vi "rotate.vi"(8 "error in (no error)":errorcluster, 10 "angle":dbl[unit], 11 "Image in":refnum<class "Image.lvclass">) -> (0 "error out":errorcluster, 3 "Image out":refnum<class "Image.lvclass">)   [LabVIEW 2010, in "Image.lvclass"]
uses:
  Image.lvclass
  storage_mode.ctl
  ErrorController/ErrorController/class_data.vi
  <vilib>/vision/NI_Vision_Development_Module.lvlib
  ErrorController/ErrorController/ErrorController.lvclass
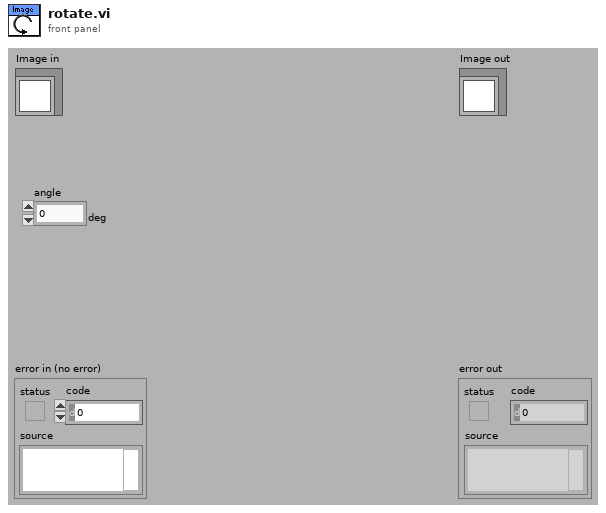
[diagram p1: front panel]
types:
  T1 = typedef "Image.lvclass/storage_mode.ctl" = enum16{"RAM", "disk"}
  T2 = typedef "IMAQ Image.ctl" = refnum<image>
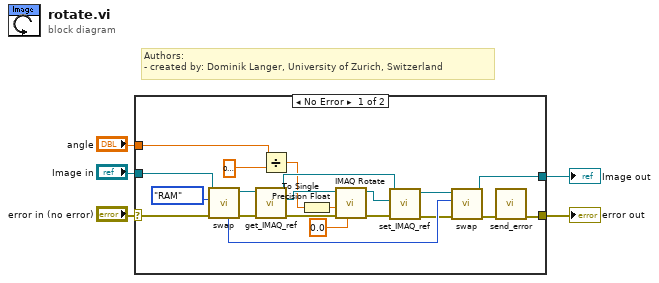
[diagram p0: block diagram]
diagram:
  # "Authors: \n- created by: Dominik Langer, University of Zurich, Switzerland"
  n1 = case shown="No Error" "error in (no error)" {
    selector: "error in (no error)" -> [w24 w28]
    tunnel: [w6 w28] -> w4
    tunnel: [w8 w27] -> w2
    tunnel: "Image in" -> [w10 w27]
    tunnel: "angle" -> [w9 _]
    frame No Error {
      n2 = call-dynamic "swap.vi"("error in (no error)"=w24, "storage type target"=storage_mode."RAM", "Image in"=w10) -> ("error out"=w23:errorcluster, "Image out"=w22:refnum<class "Image.lvclass">, "previous storage mode"=w25:T1)  [unwired: 6 out]
      n3 = call-dynamic "get_IMAQ_ref.vi"("error in (no error)"=w23, "Image.lvclass in"=w22) -> ("error out"=w21:errorcluster, "Image"=w20:T2, "Image.lvclass out"=w14:refnum<class "Image.lvclass">)  [unwired: 7 out]
      n4 = Divide(x=w9, y=dbl[unit] 0.017453292519943295 ("angle")) -> (x/y=w11:dbl)
      n5 = To Single Precision Float(number=w11) -> (single precision float=w18:sgl)
      n6 = call "IMAQ Rotate"("Replace Value"=sgl 0.0, "error in (no error)"=w21, "Angle (degrees)"=w18, "Image Src"=w20) -> ("error out"=w16:errorcluster, "Image Dst Out"=w15:T2)  [unwired: 4 in, 2 out]
      n7 = call-dynamic "set_IMAQ_ref.vi"("error in (no error)"=w16, "Image"=w15, "Image.lvclass in"=w14) -> ("error out"=w13:errorcluster, "Image.lvclass out"=w12:refnum<class "Image.lvclass">)  [unwired: 7 out]
      n8 = call-dynamic "swap.vi"("error in (no error)"=w13, "storage type target"=w25, "Image in"=w12) -> ("error out"=w7:errorcluster, "Image out"=w8:refnum<class "Image.lvclass">)  [unwired: 7 out]
      n9 = call "send_error.vi"("error in (no error)"=w7) -> ("error out"=w6:errorcluster)  [unwired: 10 in]
    }
    frame Error {
    }
  }
  "error out" <- w4
  "Image out" <- w2
